vi "Rogel_Anthony_Campues_Vicente_G2_Autotrinica.vi"() -> ()   [LabVIEW 2025]
uses:
  <vilib>/express/express arith-compare/Formula/XNode/ExpressFormulaBlockNode.xnode
panel:
  out "Celcius":dbl(slide) scale=0.0..400.0
  out "frio":bool
  out "caliente":bool
  in  "Slide":dbl(slide) scale=0.0..100.0
  out "Celcius":dbl(knob) scale=0.0..400.0
  out "Celcius":dbl
  out "KeLvin":dbl(knob) scale=0.0..400.0
  out "Fahrenheit":dbl(knob) scale=0.0..400.0
  in  "stop":bool
  out "KeLvin":dbl(knob) scale=0.0..400.0
  out "Fahrenheit":dbl(knob) scale=0.0..400.0
  out "KeLvin":dbl
  out "Fahrenheit":dbl
  out "kelvin":dbl(slide) scale=0.0..400.0
  out "Fahrenheit":dbl(slide) scale=0.0..400.0
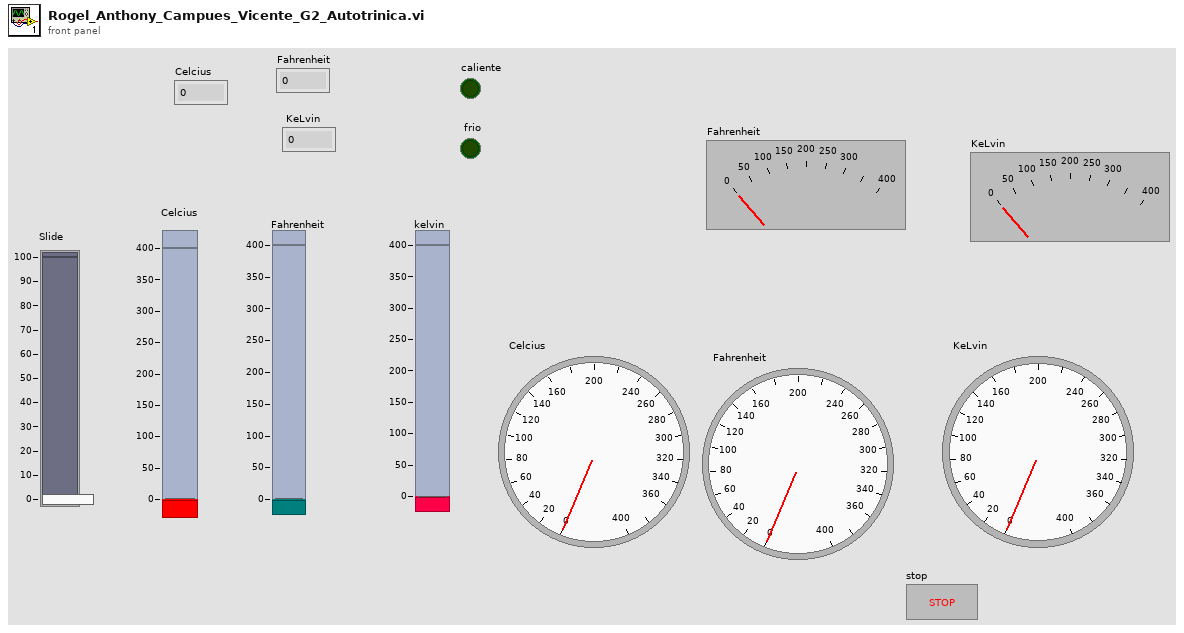
[diagram p1: front panel]
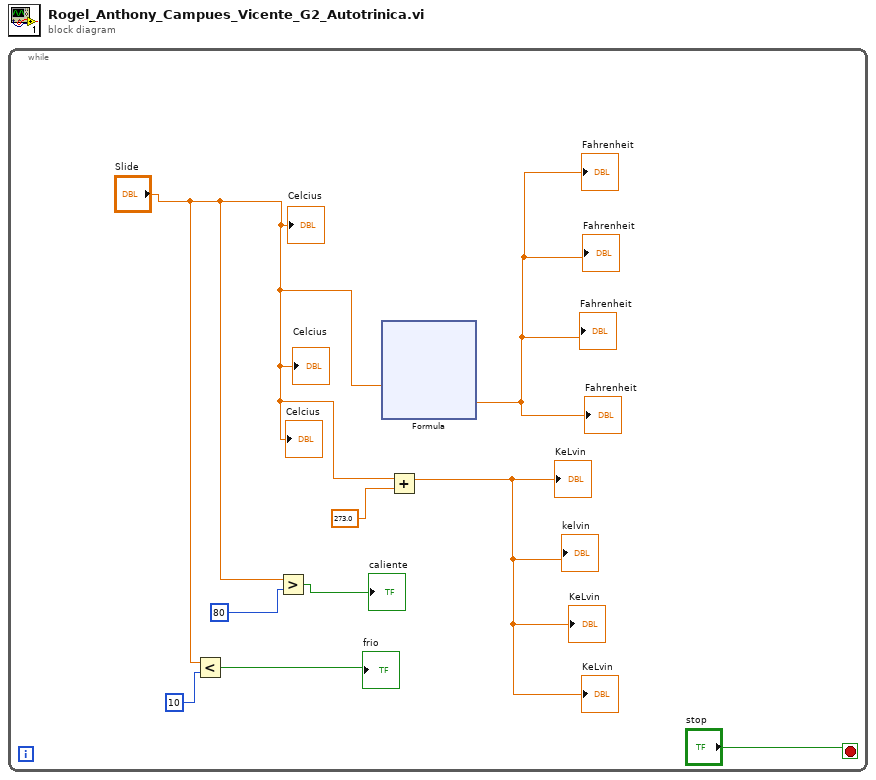
[diagram p0: block diagram]
diagram:
  n1 = while {
    stop <- "stop" stop-if-true
    n2 = Less?(x="Slide", y=10) -> (x < y?=→"frio":bool)
    n3 = Greater?(x="Slide", y=80) -> (0:→"caliente":bool)
    n4 = xnode "Formula"("X1"="Slide") -> ("Result"=→"Fahrenheit" →"Fahrenheit" →"Fahrenheit" →"Fahrenheit":dbl)  [unwired: 1 in, 1 out]
    n5 = Add(x="Slide", y=273.0) -> (x+y=→"kelvin" →"KeLvin" →"KeLvin" →"KeLvin":dbl)
    "Celcius" <- "Slide"
    "Celcius" <- "Slide"
    "Celcius" <- "Slide"
  }
